vi "SVG2VSDXBatch.vi"() -> ()   [LabVIEW 2018]
uses:
  <vilib>/TaskbarProgressAPI/_TypeDefs/Progress State.ctl
  <userlib>/_OpenG.lib/file/file.llb/Convert File Extension (Path)__ogtk.vi
  <vilib>/TaskbarProgressAPI/TaskbarProgressAPI.lvlib
panel:
  in  "转换":bool
  in  "打开":bool
  out "SVG文件数":i32
  in  "使用源路径":bool
  in  "输出格式":enum16{"VSDX", "VSD", "EMF"}(ring)
  in  "VSDX目录":path
  out "SVG目录":path
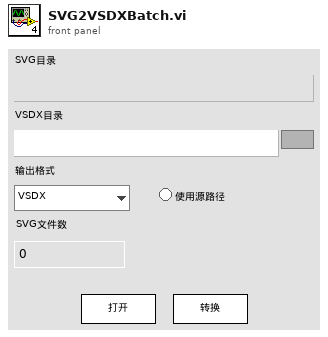
[diagram p1: front panel]
types:
  T1 = typedef "TaskbarProgressAPI.lvlib/Progress State.ctl" = i32
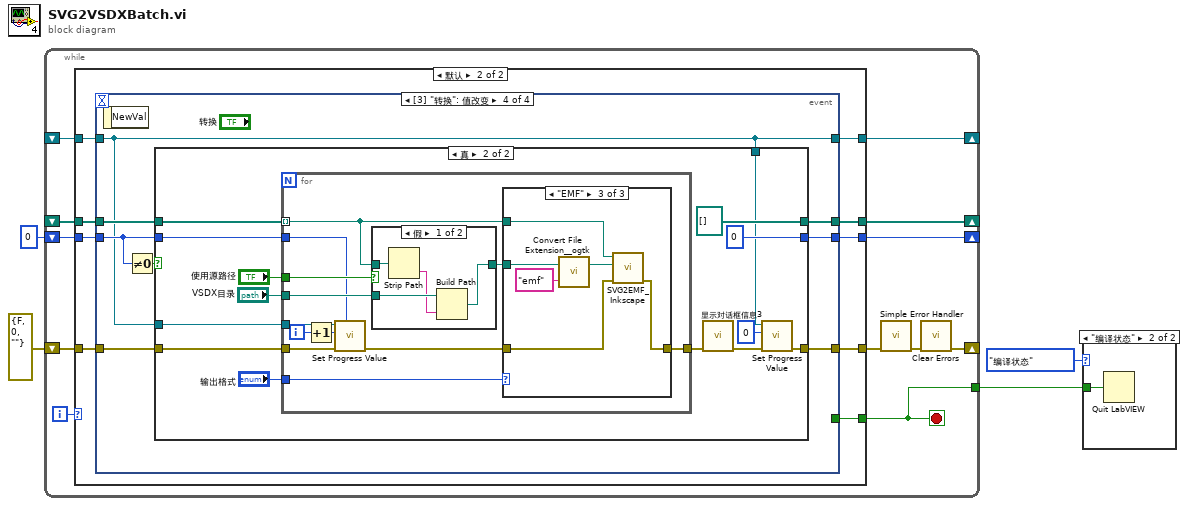
[diagram p0: block diagram]
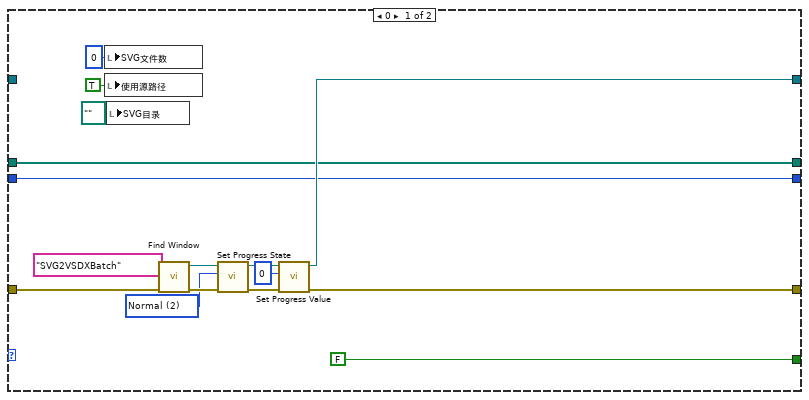
[diagram p3: hidden frame]
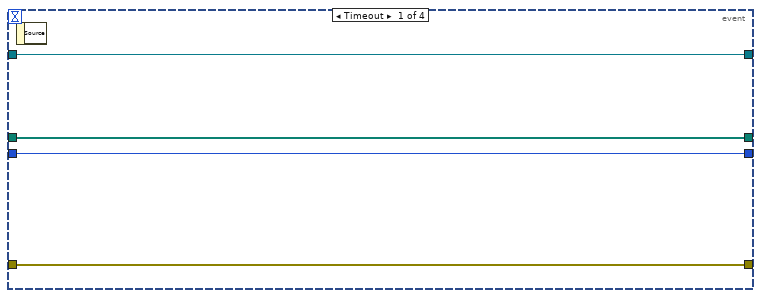
[diagram p4: hidden frame]
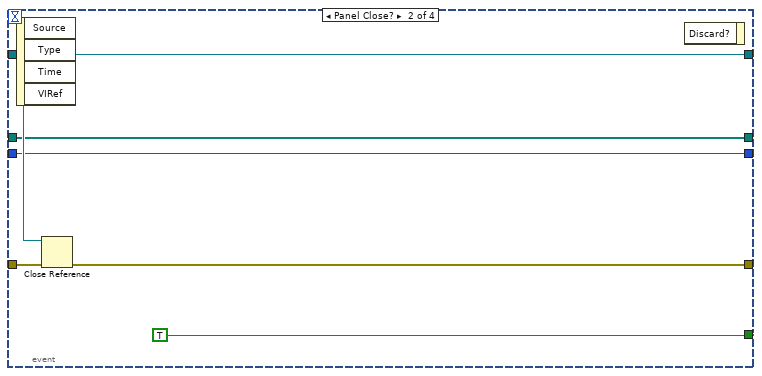
[diagram p5: hidden frame]
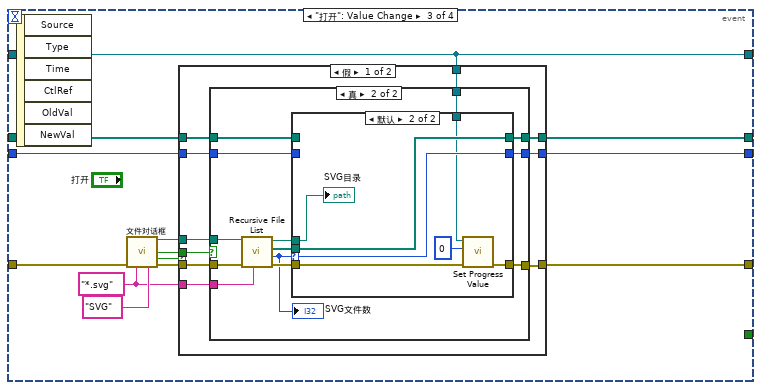
[diagram p6: hidden frame]
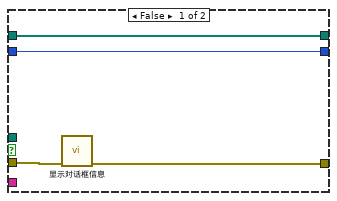
[diagram p7: hidden frame]
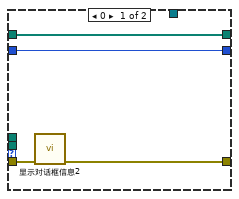
[diagram p8: hidden frame]
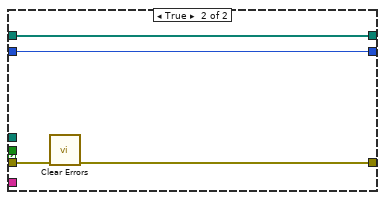
[diagram p9: hidden frame]
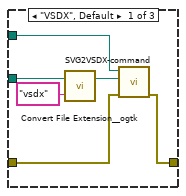
[diagram p11: hidden frame]
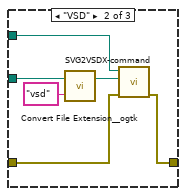
[diagram p12: hidden frame]
diagram:
  n1 = while {
    tunnel: [w11] -> w3
    shift-right: [w12] -> _
    shift-left: errorcluster {"status"=FALSE, "code"=0, "source"=""} ("错误常量") -> [w15]
    shift-right: [w10] -> _
    shift-left: _ -> [w9]
    shift-right: [w8] -> _
    shift-left: _ -> [w7]
    shift-right: [w6] -> _
    shift-left: 0 ("Number of Files") -> [w5]
    i -> [w16]
    stop <- w11 stop-if-true
    n2 = case shown="默认" w16 {
      tunnel: w15 -> [w32 w41]
      tunnel: [w22 w40] -> w14
      tunnel: [FALSE w39] -> w11
      tunnel: [w19 w37] -> w10
      tunnel: w9 -> [_ w38]
      tunnel: [w18 w36] -> w8
      tunnel: w7 -> [w18 w35]
      tunnel: [w17 w34] -> w6
      tunnel: w5 -> [w17 w33]
      frame 0 {
        w23 = T1 2 items=["NoProgress"=0, "Indeterminate"=1, "Normal"=2, "Error"=4, "Paused"=8] ("State (No Progress)")
        # "初始化"
        n3 = local write "SVG文件数"(0 ("SVG文件数")) -> ()
        n4 = local write "使用源路径"(TRUE ("使用源路径")) -> ()
        n5 = local write "SVG目录"(path "" ("SVG目录")) -> ()
        n6 = call <vilib>:"Find Window.vi"("error in (no error)"=w32, "Window Title (Callers Window)"="SVG2VSDXBatch") -> ("error out"=w27:errorcluster, "Window Handle"=w24:refnum<k24>)  [unwired: 8 in]
        n7 = call <vilib>:"Set Progress State.vi"("error in (no error)"=w27, "State (No Progress)"=w23, "Window Handle"=w24) -> ("error out"=w25:errorcluster, "dup Window Handle"=w21:refnum<k24>)  [unwired: 7 in]
        n8 = call <vilib>:"Set Progress Value.vi"("error in (no error)"=w25, "current (0)"=u64 0, "Window Handle"=w21) -> ("error out"=w22:errorcluster, "dup Window Handle"=w19:refnum<k24>)  [unwired: 7 in]
      }
      frame Default {
        n9 = event shown="[3] \"转换\": 值改变" {
          selector: _ -> [_ _ _ _]
          dyn-events: _ -> [_ _ _ _]
          timeout: _ -> [_ _ _ _]
          tunnel: w41 -> [w45 w51 w64 w111]
          tunnel: [w45 w49 w61 w110] -> w40
          tunnel: [_ TRUE _ _] -> w39
          tunnel: w38 -> [w44 w48 w53 w107]
          tunnel: [w44 w48 w53 w107] -> w37
          tunnel: [w43 w47 w56 w109] -> w36
          tunnel: w35 -> [w43 w47 w55 w114]
          tunnel: [w42 w46 w54 w108] -> w34
          tunnel: w33 -> [w42 w46 w52 w112]
          event Timeout {
            n10 = event-data() -> ()  [unwired: 1 in, 1 out]
          }
          event Panel Close? {
            n11 = event-data() -> ()  [unwired: 1 in, 4 out]
            n12 = Close Reference(reference=w48, error in (no error)=w51) -> (error out=w49:errorcluster)
            n13 = event-data() -> ()  [unwired: 2 in, 1 out]
          }
          event "打开": Value Change {
            w57 = "*.svg" ("pattern (all files)")
            n14 = event-data() -> ()  [unwired: 1 in, 6 out]
            n15 = call "文件对话框"("error in"=w64, "pattern (all files)"=w57, "pattern label"="SVG") -> ("selected path"=w58:path, "exists"=w59:bool, "cancelled"=w60:bool, "error out"=w63:errorcluster)  [unwired: 9 in]
            n16 = case shown="假" w60 {
              tunnel: w63 -> [w73 w106]
              tunnel: [w72 w105] -> w61
              tunnel: w59 -> [w74 _]
              tunnel: w58 -> [w71 _]
              tunnel: w57 -> [w70 _]
              tunnel: [w69 w104] -> w56
              tunnel: w55 -> [w68 w104]
              tunnel: [w67 w103] -> w54
              tunnel: w53 -> [w66 _]
              tunnel: w52 -> [w65 w103]
              frame False {
                n17 = case shown="真" w74 {
                  tunnel: w73 -> [w78 w91]
                  tunnel: [w77 w87] -> w72
                  tunnel: w71 -> [_ w89]
                  tunnel: w70 -> [_ w88]
                  tunnel: [w76 w85] -> w69
                  tunnel: w68 -> [w76 w84]
                  tunnel: [w75 w82] -> w67
                  tunnel: w66 -> [_ w81]
                  tunnel: w65 -> [w75 w80]
                  frame False {
                    n18 = call "显示对话框信息"("error in (no error)"=w78) -> ("error out"=w77:errorcluster)  [unwired: 9 in, 1 out]
                  }
                  frame True {
                    n19 = call <vilib>:"Recursive File List.vi"("pattern"=w88, "error in (no error)"=w91, "Folder Path"=w89) -> ("error out"=w90:errorcluster, "Number of Files"=w83:i32, "All Files in Dir"=w86:path[], "dup Folder Path"=w79:path)  [unwired: 4 in, 1 out]
                    "SVG文件数" <- w83
                    n20 = case shown="默认" w83 {
                      selector: w83 -> [_ w99]
                      tunnel: w90 -> [w95 w102]
                      tunnel: [w94 w100] -> w87
                      tunnel: w86 -> [_ w101]
                      tunnel: [w93 w101] -> w85
                      tunnel: w84 -> [w93 _]
                      tunnel: [w92 w99] -> w82
                      tunnel: w81 -> [_ w97]
                      tunnel: w80 -> [w92 _]
                      tunnel: w79 -> [_ w96]
                      frame 0 {
                        n21 = call "显示对话框信息2"("error in (no error)"=w95) -> ("error out"=w94:errorcluster)  [unwired: 9 in, 1 out]
                      }
                      frame Default {
                        n22 = call <vilib>:"Set Progress Value.vi"("error in (no error)"=w102, "current (0)"=u64 0, "Window Handle"=w97) -> ("error out"=w100:errorcluster)  [unwired: 7 in, 1 out]
                        "SVG目录" <- w96
                      }
                    }
                  }
                }
              }
              frame True {
                n23 = call <vilib>:"Clear Errors.vi"("error in (no error)"=w106) -> ("error out"=w105:errorcluster)  [unwired: 5 in, 1 out]
              }
            }
          }
          event "转换": Value Change {
            n24 = event-data() -> ()  [unwired: 1 in, 1 out]
            n25 = Not Equal To 0?(x=w112) -> (x != 0?=w113:bool)
            n26 = case shown="真" w113 {
              tunnel: w114 -> [w117 w131]
              tunnel: w112 -> [w116 w122]
              tunnel: w111 -> [w115 w127]
              tunnel: [w115 w120] -> w110
              tunnel: [w117 path[] [] ("All Files in Dir")] -> w109
              tunnel: [w116 0] -> w108
              tunnel: w107 -> [_ w121]
              tunnel: w107 -> [_ w119]
              frame False {
              }
              frame True {
                n27 = for {
                  tunnel: w131 -> [w140] mode=indexing
                  tunnel: "使用源路径" -> [w143]
                  tunnel: "VSDX目录" -> [w142]
                  tunnel: "输出格式" -> [w134]
                  tunnel: w127 -> [w139]
                  tunnel: [w138] -> w126
                  tunnel: w122 -> [w136]
                  tunnel: w121 -> [w135]
                  i -> [w132]
                  n28 = Increment(x=w132) -> (x+1=w133:i32)
                  n29 = call <vilib>:"Set Progress Value.vi"("maximum (100)"=w136, "error in (no error)"=w139, "current (0)"=w133, "Window Handle"=w135) -> ("error out"=w137:errorcluster)  [unwired: 6 in, 1 out]
                  n30 = case shown="假" w143 {
                    tunnel: w140 -> [w165 w166]
                    tunnel: w142 -> [w164 _]
                    tunnel: [w162 w166] -> w141
                    frame False {
                      n31 = Strip Path(path=w165) -> (name=w163:string)  [unwired: 1 out]
                      n32 = Build Path(base path=w164, name or relative path=w163) -> (appended path=w162:path)
                    }
                    frame True {
                    }
                  }
                  n33 = case shown="\"EMF\"" w134 {
                    tunnel: w141 -> [w149 w155 w161]
                    tunnel: w140 -> [w147 w153 w159]
                    tunnel: w137 -> [w145 w151 w157]
                    tunnel: [w144 w150 w156] -> w138
                    frame "VSDX", Default {
                      n34 = call-poly <userlib>:"Convert File Extension__ogtk.vi"("new ending (none)"="vsdx", "file name"=w149) -> ("new filename"=w146:path)  [unwired: 1 out]
                      n35 = call "SVG2VSDX-command.vi"("Error in"=w145, "vsd路径"=w146, "svg路径"=w147) -> ("Error out"=w144:errorcluster)  [unwired: 8 in]
                    }
                    frame "VSD" {
                      n36 = call-poly <userlib>:"Convert File Extension__ogtk.vi"("new ending (none)"="vsd", "file name"=w155) -> ("new filename"=w152:path)  [unwired: 1 out]
                      n37 = call "SVG2VSDX-command.vi"("Error in"=w151, "vsd路径"=w152, "svg路径"=w153) -> ("Error out"=w150:errorcluster)  [unwired: 8 in]
                    }
                    frame "EMF" {
                      n38 = call-poly <userlib>:"Convert File Extension__ogtk.vi"("new ending (none)"="emf", "file name"=w161) -> ("new filename"=w158:path)  [unwired: 1 out]
                      n39 = call "SVG2EMF_Inkscape.vi"("error in"=w157, "emf路径"=w158, "svg路径"=w159) -> ("error out"=w156:errorcluster)  [unwired: 7 in, 1 out]
                    }
                  }
                }
                n40 = call "显示对话框信息3"("error in (no error)"=w126) -> ("error out"=w125:errorcluster)  [unwired: 9 in, 1 out]
                n41 = call <vilib>:"Set Progress Value.vi"("error in (no error)"=w125, "current (0)"=u64 0, "Window Handle"=w119) -> ("error out"=w120:errorcluster)  [unwired: 7 in, 1 out]
              }
            }
          }
        }
      }
    }
    n42 = call <vilib>:"Simple Error Handler.vi"("error in (no error)"=w14) -> ("error out"=w13:errorcluster)  [unwired: 4 in, 4 out]
    n43 = call <vilib>:"Clear Errors.vi"("error in (no error)"=w13) -> ("error out"=w12:errorcluster)  [unwired: 5 in, 1 out]
  }
  n44 = case shown="\"编译状态\"" enum16{"设计状态", "编译状态"}."编译状态" {
    tunnel: w3 -> [_ w167]
    frame "设计状态", Default {
    }
    frame "编译状态" {
      n45 = Quit LabVIEW(quit? (T)=w167) -> ()
    }
  }
